vi "Create Array (SubVI).vi"(11 "Sample quantity in":i32=64) -> (1 "Sample quantity out":i32, 2 "Array":i32[](array[numeric]), 3 "Array 2":i32[](array[numeric]))   [LabVIEW 2012]
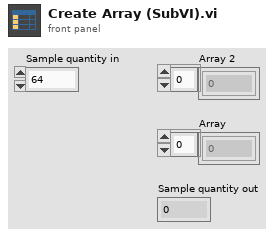
[diagram p1: front panel]
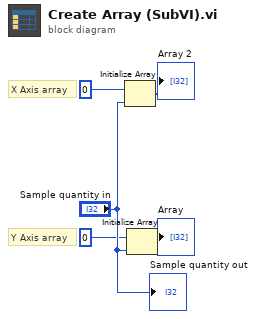
[diagram p0: block diagram]
diagram:
  # "Y Axis array"
  # "X Axis array"
  n1 = Initialize Array(0 ("element"), "Sample quantity in") -> (→"Array 2":i32[])
  n2 = Initialize Array(0 ("element"), "Sample quantity in") -> (→"Array":i32[])
  "Sample quantity out" <- "Sample quantity in"
